vi "Parse GXML.vi"() -> ()   [LabVIEW 2009]
doc: "This example demonstrates how to convert an XML string into a LabVIEW data structure using the GXML reference library."
uses:
  _subVIis/GXML Quick Parser/gxml_QuickParser.vi
panel:
  in  "Read XML from File?":bool
  out "Cont1_Cluster":T1={"Cont2_Array"=[[{"Cal"=TRUE, "Cont4_Cluster"={"Samps"=5, "Cont5_Array"=[[-5.1, -2.1], [-4.1, -1.1], [-3.1, -0.1]]}}, {"Cal"=FALSE, "Cont4_Cluster"={"Samps"=16, "Cont5_Array"=[]}}, {"Cal"=FALSE, "Cont4_Cluster"={"Samps"=24, "Cont5_Array"=[[0.0, 2.0], [1.0, 1.0], [2.0, 0.0]]}}, {"Cal"=TRUE, "Cont4_Cluster"={"Samps"=38, "Cont5_Array"=[[123.456, 456.123], [234.561, 561.234], [345.612, 612.345]]}}]], "X.Axis.Pos"=16.5-2.3i, "Enum3D_Array"=[[[enum."See", enum."Spot", enum."Run"], [enum."Run", enum."Spot", enum."Run"]], [[enum."See", enum."Spot", enum."Jump"], [enum."Jump", enum."Spot", enum."Jump"]]], "Text Cluster"={"Msg_Array"=["Hello", "World"], "Path_Array"=[path "C:/File Main", path "D:/Jeff"]}, "Trigger_Times"=[timestamp(3340037987.3199577 s since 1904-01-01), timestamp(3340642787.3199577 s since 1904-01-01), timestamp(3341247587.3199577 s since 1904-01-01)], "Description"={"Description"=["Life", "Universe", "Everything"], "FinalCfg"=enum."Larry"}}
  in  "XML String Out":string="<GXML_Root>\r\n  <Cont1_Cluster mems='6'>\r\n    <Cont2_Array dim='[1,4]' type='Cluster'>\r\n      <Cont3_Cluster mems='2'>\r\n        <Cal type='Bool'>TRUE</Cal>\r\n        <Cont4_Cluster mems='2'>\r\n          <Samps type='U32'>5</Samps>\r\n          <Cont5_Array dim='[3,2]' type='SGL'>\r\n            <Gain>-5.1</Gain>\r\n            <Gain>-2.1</Gain>\r\n            <Gain>-4.1</Gain>\r\n            <Gain>-1.1</Gain>\r\n            <Gain>-3.1</Gain>\r\n            <Gain>-0.1</Gain>\r\n          </Cont5_Array>\r\n        </Cont4_Cluster>\r\n      </Cont3_Cluster>\r\n      <Cont3_Cluster mems='2'>\r\n        <Cal type='Bool'>FALSE</Cal>\r\n        <Cont4_Cluster mems='2'>\r\n          <Samps type='U32'>16</Samps>\r\n          <Cont5_Array dim='[0,0]' type='SGL'>\r\n            <Gain></Gain>\r\n          </Cont5_Array>\r\n        </Cont4_Cluster>\r\n      </Cont3_Cluster>\r\n      <Cont3_Cluster mems='2'>\r\n        <Cal type='Bool'>FALSE</Cal>\r\n        <Cont4_Cluster mems='2'>\r\n          <Samps type='U32'>24</Samps>\r\n          <Cont5_Array dim='[3,2]' type='SGL'>\r\n            <Gain>0</Gain>\r\n            <Gain>2</Gain>\r\n            <Gain>1</Gain>\r\n            <Gain>1</Gain>\r\n            <Gain>2</Gain>\r\n            <Gain>0</Gain>\r\n          </Cont5_Array>\r\n        </Cont4_Cluster>\r\n      </Cont3_Cluster>\r\n      <Cont3_Cluster mems='2'>\r\n        <Cal type='Bool'>TRUE</Cal>\r\n        <Cont4_Cluster mems='2'>\r\n          <Samps type='U32'>38</Samps>\r\n          <Cont5_Array dim='[3,2]' type='SGL'>\r\n            <Gain>123.456001</Gain>\r\n            <Gain>456.122986</Gain>\r\n            <Gain>234.561005</Gain>\r\n            <Gain>561.234009</Gain>\r\n            <Gain>345.612</Gain>\r\n            <Gain>612.344971</Gain>\r\n          </Cont5_Array>\r\n        </Cont4_Cluster>\r\n      </Cont3_Cluster>\r\n    </Cont2_Array>\r\n    <X.Axis.Pos type='CXT'>16.5 -2.3 i</X.Axis.Pos>\r\n    <Enum3D_Array dim='[2,2,3]' type='Enum U16'>\r\n      <MarkEnum sel='See'>0</MarkEnum>\r\n      <MarkEnum sel='Spot'>1</MarkEnum>\r\n      <MarkEnum sel='Run'>2</MarkEnum>\r\n      <MarkEnum sel='Run'>2</MarkEnum>\r\n      <MarkEnum sel='Spot'>1</MarkEnum>\r\n      <MarkEnum sel='Run'>2</MarkEnum>\r\n      <MarkEnum sel='See'>0</MarkEnum>\r\n      <MarkEnum sel='Spot'>1</MarkEnum>\r\n      <MarkEnum sel='Jump'>3</MarkEnum>\r\n      <MarkEnum sel='Jump'>3</MarkEnum>\r\n      <MarkEnum sel='Spot'>1</MarkEnum>\r\n      <MarkEnum sel='Jump'>3</MarkEnum>\r\n    </Enum3D_Array>\r\n    <Text_Cluster mems='2'>\r\n      <Msg_Array dim='[2]' type='String'>\r\n        <Msg>Hello</Msg>\r\n        <Msg>World</Msg>\r\n      </Msg_Array>\r\n      <Path_Array dim='[2]' type='Path'>\r\n        <Cfg_File>C:\\File Main</Cfg_File>\r\n        <Cfg_File>D:\\Jeff</Cfg_File>\r\n      </Path_Array>\r\n    </Text_Cluster>\r\n    <Trigger_Times dim='[3]' type='Time'>\r\n      <Start>14:19:47 11/2/2009</Start>\r\n      <Start>14:19:47 11/9/2009</Start>\r\n      <Start>14:19:47 11/16/2009</Start>\r\n    </Trigger_Times>\r\n    <Description mems='2'>\r\n      <Description dim='[3]' type='String'>\r\n        <Description>Life</Description>\r\n        <Description>Universe</Description>\r\n        <Description>Everything</Description>\r\n      </Description>\r\n      <FinalCfg type='Enum U8' sel='Larry'>0</FinalCfg>\r\n    </Description>\r\n  </Cont1_Cluster>\r\n</GXML_Root>"
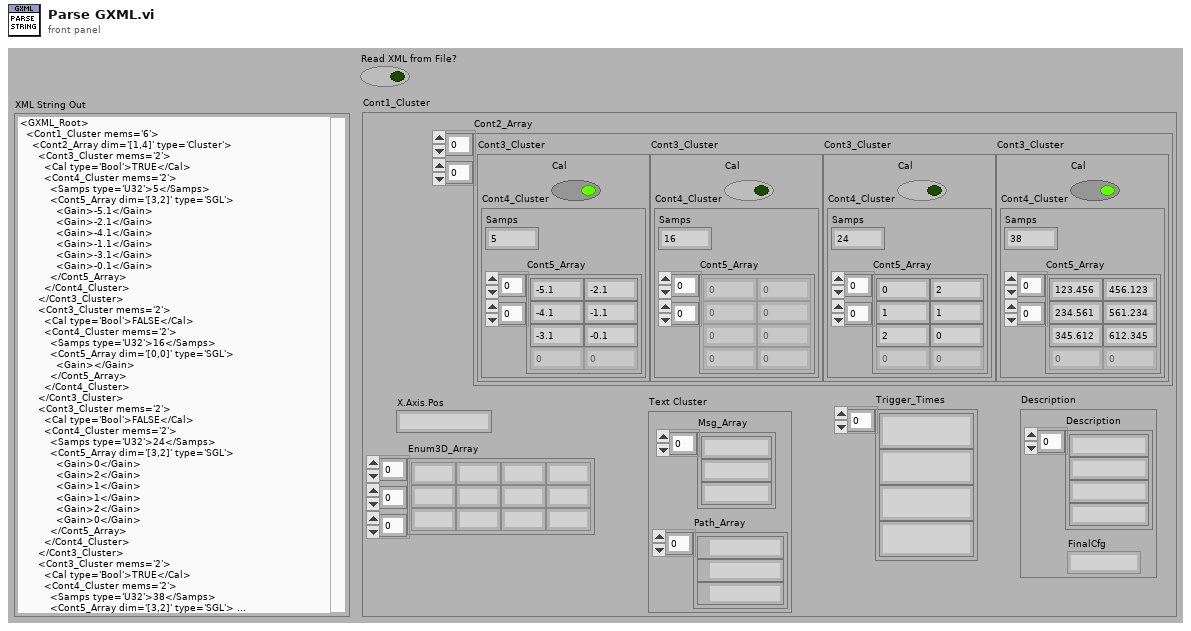
[diagram p1: front panel]
types:
  T1 = cluster{"Cont2_Array":cluster{"Cal":bool, "Cont4_Cluster":cluster{"Samps":u32, "Cont5_Array":sgl[][]}}[][], "X.Axis.Pos":cxt, "Enum3D_Array":enum16{"See", "Spot", "Run", "Jump"}[][][], "Text Cluster":cluster{"Msg_Array":string[], "Path_Array":path[]}, "Trigger_Times":timestamp[], "Description":cluster{"Description":string[], "FinalCfg":enum8{"Larry", "Curly", "Moe"}}}
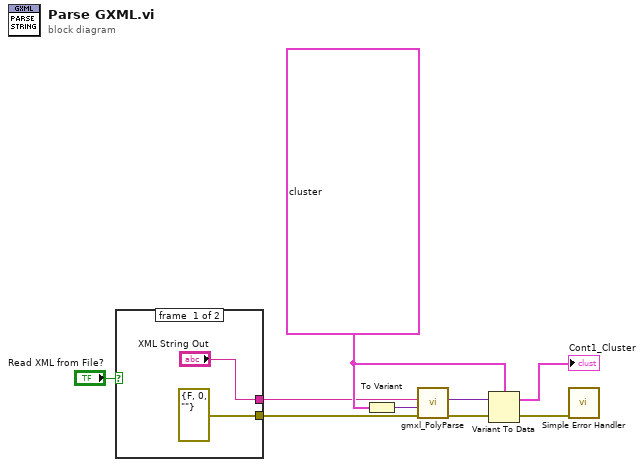
[diagram p0: block diagram]
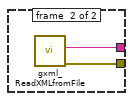
[diagram p2: hidden frame]
diagram:
  w5 = T1 {"Cont2_Array"=[], "X.Axis.Pos"=0.0+0.0i, "Enum3D_Array"=[], "Text Cluster"={"Msg_Array"=[], "Path_Array"=[]}, "Trigger_Times"=[], "Description"={"Description"=[], "FinalCfg"=enum."Larry"}} ("Cont1_Cluster")
  n1 = case shown="True" "Read XML from File?" {
    tunnel: [errorcluster {"status"=FALSE, "code"=0, "source"=""} ("error out") w13] -> w2
    tunnel: ["XML String Out" w12] -> w1
    frame #0 {
    }
    frame #1 {
      n2 = call "gxml_ReadXMLfromFile.vi"() -> ("error out"=w13:errorcluster, "XML String Out"=w12:string)  [unwired: 9 in, 1 out]
    }
  }
  n3 = To Variant(anything=w5) -> (Variant=w6:variant)
  n4 = call-poly "gmxl_PolyParse.vi"("error in (no error)"=w2, "TypeDesc"=w6, "XML File String"=w1) -> ("error out"=w9:errorcluster, "Parsed Data"=w8:variant)  [unwired: 7 in]
  n5 = Variant To Data(error in=w9, Variant=w8, type=w5) -> (error out=w7:errorcluster, data=→"Cont1_Cluster":T1)
  n6 = call <vilib>:"Simple Error Handler.vi"("error in (no error)"=w7) -> ()  [unwired: 4 in, 5 out]
